vi "Elements by Indices.vi"(8 "error in (no error)":errorcluster, 9 "Indices":i32[](array[numeric]), 11 "Config Manager in":refnum<class "Config Manager.lvclass">) -> (0 "error out":errorcluster, 2 "Elements":refnum<class "Config Element.lvclass">[](array[class]), 3 "Config Manager out":refnum<class "Config Manager.lvclass">)   [LabVIEW 2020, in "CDM-Config.lvlib" / "Config Manager.lvclass"]
uses:
  Config Manager.lvclass
  Config Element/Config Element.lvclass
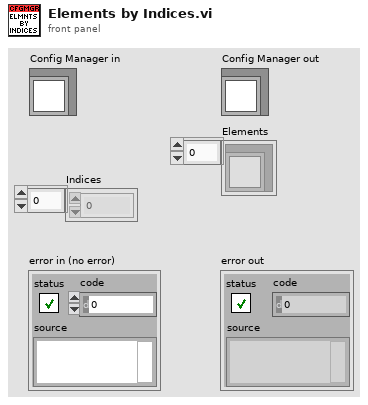
[diagram p1: front panel]
types:
  T1 = typedef "CDM-Config.lvlib/Config Manager.lvclass/Ref Data.ctl" = cluster{"Elements":refnum<class "Config Element.lvclass">[], "Hierarchy Map":map{string[], i32}, "Element Map":map{refnum<class "Config Element.lvclass">, i32}}
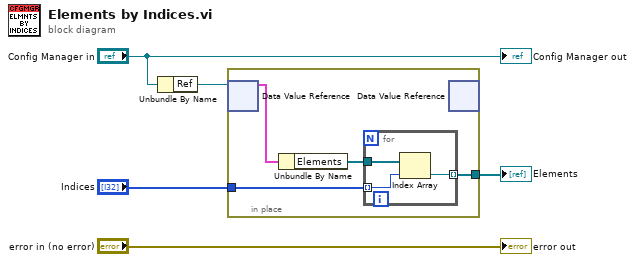
[diagram p0: block diagram]
diagram:
  n1 = Unbundle By Name("Config Manager in") -> ("Ref"=w4:refnum<data-value>)
  n2 = in-place {
    in-place-border: [w7] -> w2
    in-place-border: "Indices" -> [w6]
    n3 = in-place-dvr #1(w4) -> (w9:T1)  [unwired: 1 out]
    n4 = Unbundle By Name(w9) -> ("Elements"=w8:refnum<class "Config Element.lvclass">[])
    n5 = for {
      tunnel: w8 -> [w12]
      tunnel: [w11] -> w7 mode=indexing
      tunnel: w6 -> [w10] mode=indexing
      n6 = Index Array(array=w12, index=w10) -> (element=w11:refnum<class "Config Element.lvclass">)
    }
    n7 = in-place-dvr #1() -> ()  [unwired: 1 in, 2 out]
  }
  "Elements" <- w2
  "error out" <- "error in (no error)"
  "Config Manager out" <- "Config Manager in"
